vi "例4-23.vi"() -> ()   [LabVIEW 2019]
panel:
  out "波形图":dbl[](graph)
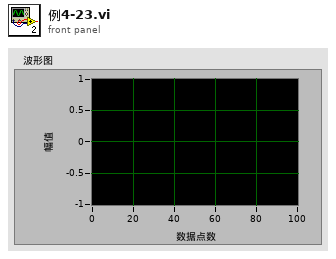
[diagram p1: front panel]
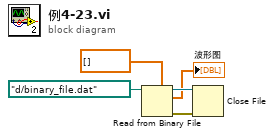
[diagram p0: block diagram]
diagram:
  n1 = Read from Binary File(5:dbl[] [], 11:path "d:/binary_file.dat" ("文件（使用对话框）")) -> (0:w2:errorcluster, 2:→"波形图":dbl[], 3:w3:refnum<file>)  [unwired: 4 in, 1 out]
  n2 = Close File(refnum=w3, error in=w2) -> ()  [unwired: 2 out]
